vi "Create Exp_tmp_reference.vi"(8 "error in (no error)":errorcluster, 11 "Control-Client in":refnum<class "Control-Client.lvclass">) -> (0 "error out":errorcluster, 3 "Control-Client out":refnum<class "Control-Client.lvclass">)   [LabVIEW 2018, in "Control-Client.lvclass"]
uses:
  Control-Client.lvclass
  Experiments/Experiment.lvclass
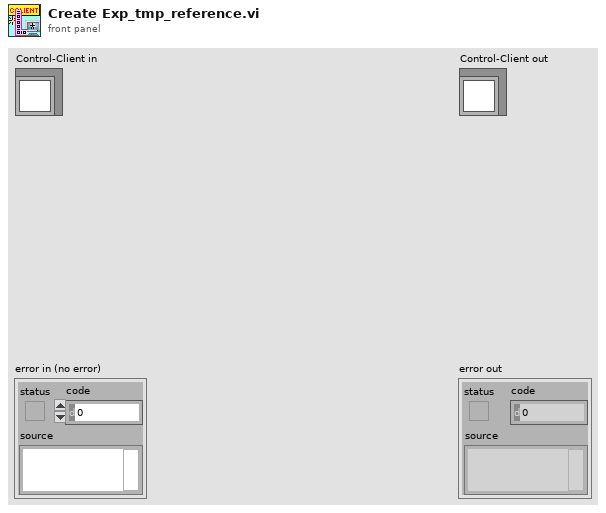
[diagram p1: front panel]
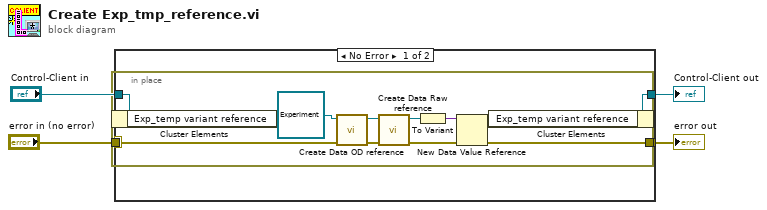
[diagram p0: block diagram]
diagram:
  n1 = case shown="No Error" "error in (no error)" {
    selector: "error in (no error)" -> [w5 w19]
    tunnel: [w6 w19] -> w3
    tunnel: [w7 w18] -> w1
    tunnel: "Control-Client in" -> [w8 w18]
    frame No Error {
      n2 = in-place {
        in-place-border: [w16] -> w6
        in-place-border: w5 -> [w14]
        n3 = in-place-cluster #1(w8) -> ()  [unwired: 1 out]
        n4 = call "Create Data OD reference.vi"("error in (no error)"=w14, "Experiment in"=refnum<class "Experiment.lvclass"> refnum ("Experiment.lvclass")) -> ("error out"=w11:errorcluster, "Experiment out"=w12:refnum<class "Experiment.lvclass">)  [unwired: 8 in]
        n5 = call "Create Data Raw reference.vi"("error in (no error)"=w11, "Experiment in"=w12) -> ("error out"=w9:errorcluster, "Experiment out"=w10:refnum<class "Experiment.lvclass">)  [unwired: 8 in]
        n6 = To Variant(anything=w10) -> (Variant=w15:variant)
        n7 = New Data Value Reference(data value=w15, error in=w9) -> (data value reference=w17:refnum<data-value>, error out=w16:errorcluster)
        n8 = in-place-cluster #1("Exp_temp variant reference"=w17) -> (w7:refnum<class "Control-Client.lvclass">)
      }
    }
    frame Error {
    }
  }
  "error out" <- w3
  "Control-Client out" <- w1
